vi "Diagrama no Labview.vi"() -> ()   [LabVIEW 2018]
uses:
  <vilib>/express/express analysis/Spectral/Block/exnSpectralBlock spectral measurements RMS poly.vi
  <vilib>/express/express analysis/Spectral/XNode/ExpressSpectralMeasurementsBlockNode.xnode
  <vilib>/express/express analysis/Spectral/Block/exnSpectralBlock spectral measurements RMS DDT.vi
panel:
  in  "A 2":dbl
  in  "F 2":dbl
  in  "A 1":dbl
  in  "F 1":dbl
  out "Dominio Da Freq":dynamicdata(graph)
  out "Dominio No Tempo":dynamicdata(graph)
  out "Duas Freq Distintas":dynamicdata(graph)
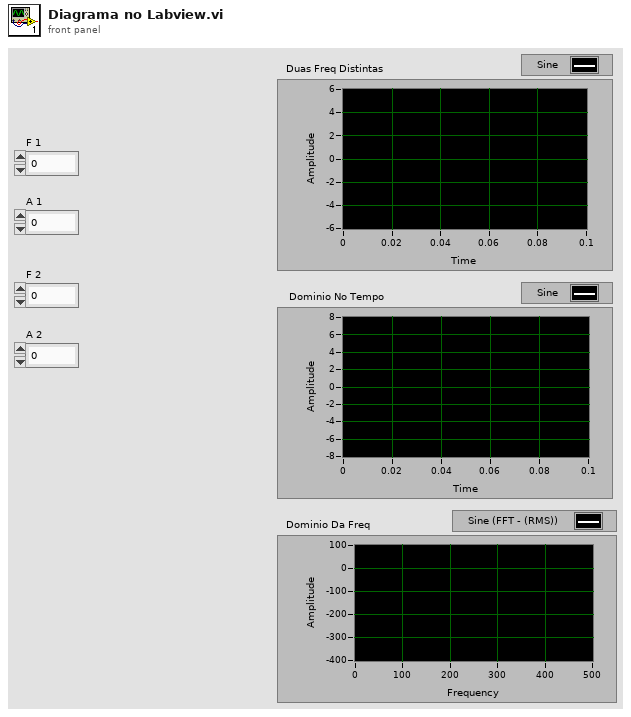
[diagram p1: front panel]
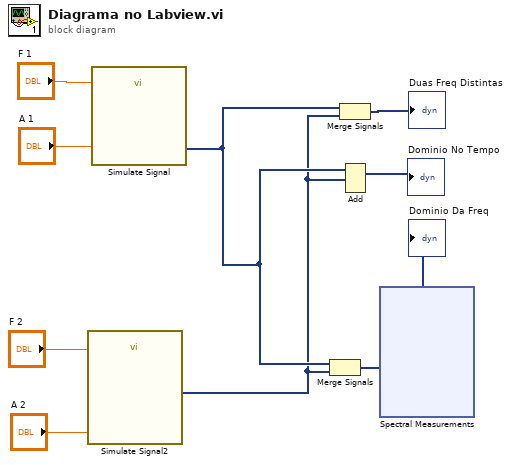
[diagram p0: block diagram]
diagram:
  n1 = call "Simulate Signal2"("Frequency"="F 2", "Amplitude"="A 2") -> ("Sine"=w2:dynamicdata)  [unwired: 12 in, 1 out]
  n2 = call "Simulate Signal"("Frequency"="F 1", "Amplitude"="A 1") -> ("Sine"=w4:dynamicdata)  [unwired: 12 in, 1 out]
  n3 = Merge Signals(w4, w2) -> (w3:dynamicdata)
  n4 = Merge Signals(w4, w2) -> (→"Duas Freq Distintas":dynamicdata)
  n5 = Add(1:w2, 2:w4) -> (0:→"Dominio No Tempo":dynamicdata)  [unwired: 1 in, 1 out]
  n6 = xnode "Spectral Measurements"("Signals"=w3) -> ("FFT - (RMS)"=→"Dominio Da Freq":dynamicdata)  [unwired: 1 in, 2 out]
